vi "Read Input DBL Values.vi"(8 "error in (no error)":errorcluster, 9 "number of registers":u16, 10 "starting address":u16, 11 "Master CR in":refnum<class "WebSocket Client CR.lvclass">) -> (0 "error out":errorcluster, 2 "data":dbl[](array[numeric]), 3 "Master CR out":refnum<class "WebSocket Client CR.lvclass">)   [LabVIEW 2021]
doc: "Reads N input registers from the device model, starting at register M."
uses:
  WebSocket Client CR.lvclass
  WebSocket Client CR.lvclass/WebSocket Client CR.ctl
  Modbus_v121c/Data Model/Device Data Model.lvclass
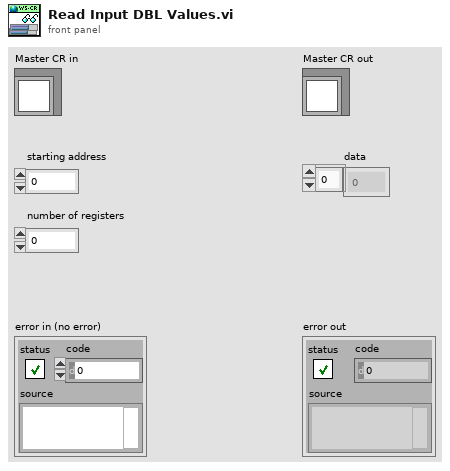
[diagram p1: front panel]
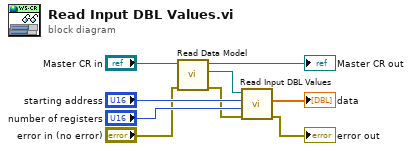
[diagram p0: block diagram]
diagram:
  n1 = call "Read Data Model.vi"("error in (no error)"="error in (no error)", "Master CR in"="Master CR in") -> ("error out"=w5:errorcluster, "Data Model"=w8:refnum<class "Device Data Model.lvclass">, "Master CR out"=→"Master CR out":refnum<class "WebSocket Client CR.lvclass">)  [unwired: 7 in]
  n2 = call-dynamic "Read Input DBL Values.vi"("error in (no error)"=w5, "number of registers"="number of registers", "starting address"="starting address", "device data model in"=w8) -> ("error out"=→"error out":errorcluster, "data"=→"data":dbl[])  [unwired: 5 in, 1 out]
